vi "Format data to plot.vi"(8 "Data Array 2":dbl[][](array[numeric]), 11 "Data Array":dbl[][](array[numeric])) -> (3 "JV Curve":cluster{"Y":dbl[], "Y":dbl[]}[](graph))   [LabVIEW 2011]
panel:
  in  "Tab Control 4":enum32{"Page 1"}(tab)
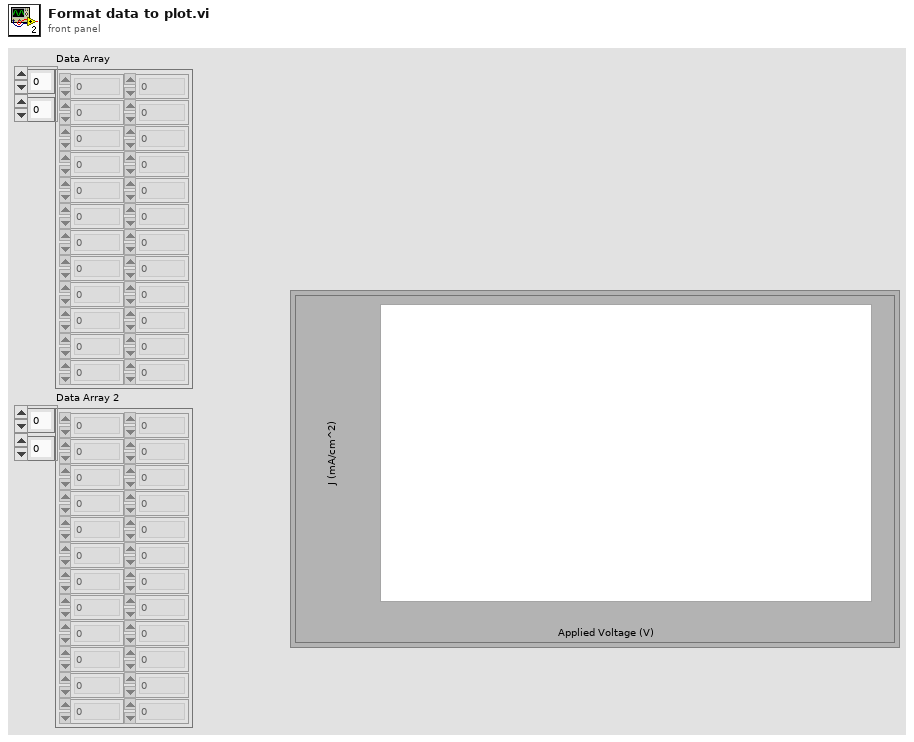
[diagram p1: front panel]
types:
  T1 = cluster{"Data Array 2":dbl[], "Data Array 2":dbl[]}
  T2 = cluster{"Data Array 2":dbl[], "Data Array 2":dbl[]}[]
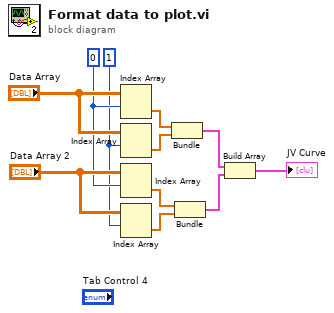
[diagram p0: block diagram]
diagram:
  w2 = 1
  w3 = 0
  n1 = Index Array(array="Data Array", index (row)=w3) -> (element=w9:dbl[])  [unwired: 1 in]
  n2 = Index Array(array="Data Array", index (row)=w2) -> (element=w8:dbl[])  [unwired: 1 in]
  n3 = Index Array(array="Data Array 2", index (row)=w3) -> (element=w7:dbl[])  [unwired: 1 in]
  n4 = Index Array(array="Data Array 2", index (row)=w2) -> (element=w6:dbl[])  [unwired: 1 in]
  n5 = Bundle("Data Array"=w9, "Data Array"=w8) -> (w4:cluster{"Data Array":dbl[], "Data Array":dbl[]})  [unwired: 1 in]
  n6 = Bundle("Data Array 2"=w7, "Data Array 2"=w6) -> (w5:T1)  [unwired: 1 in]
  n7 = Build Array(w4, w5) -> (→"JV Curve":T2)
